vi "binary to msgpack.vi"(11 "binary":u8[](array[numeric])) -> (3 "msgpack":u8[](array[numeric]) format="%x")   [LabVIEW 2020, in "MessagePack.lvlib" / "MessagePack.lvclass"]
uses:
  MessagePack.lvclass
  MessagePack.lvclass/MessagePack.ctl
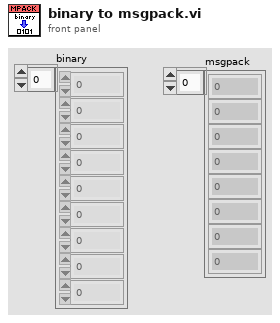
[diagram p1: front panel]
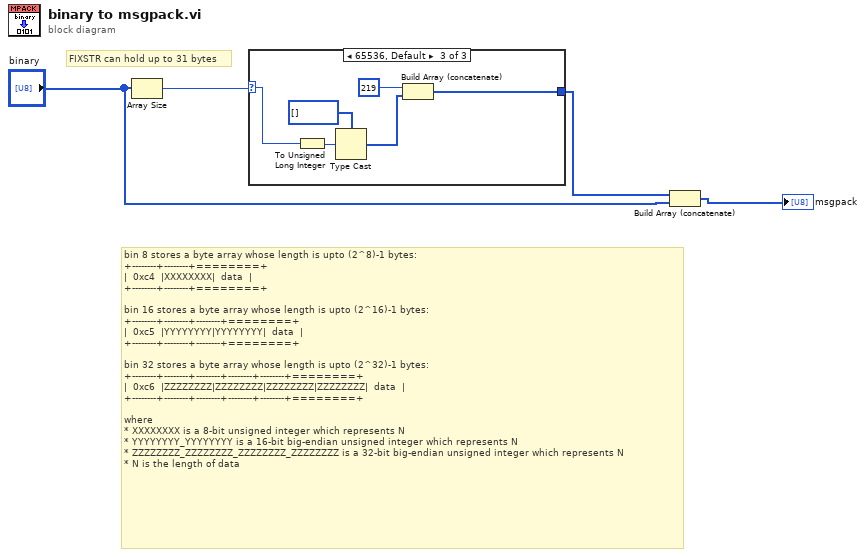
[diagram p0: block diagram]
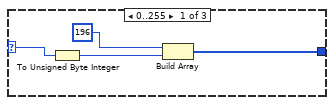
[diagram p2: hidden frame]
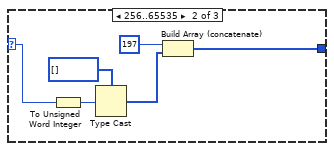
[diagram p3: hidden frame]
diagram:
  # "bin 8 stores a byte array whose length is upto (2^8)-1 bytes:\n+--------+--------+========+\n|  0xc4  |XXXXXXXX|  data  |\n+--------+--------+========+\n\nbin 16 stores a byte array whose length is upto (2^16)-1 bytes:\n+--------+--------+--------+========+\n|  0xc5  |YYYYYYYY|YYYYYYYY|  data  |\n+--------+--------+--------+========+\n\nbin 32 stores a byte array whose length is upto (2^32)-1 bytes:\n+--------+--------+--------+--------+--------+========+\n|  0xc6  |ZZZZZZZZ|ZZZZZZZZ|ZZZZZZZZ|ZZZZZZZZ|  data  |\n+--------+--------+--------+--------+--------+========+\n\nwhere\n* XXXXXXXX is a 8-bit unsigned integer which represents N\n* YYYYYYYY_YYYYYYYY is a 16-bit big-endian unsigned integer which represents N\n* ZZZZZZZZ_ZZZZZZZZ_ZZZZZZZZ_ZZZZZZZZ is a 32-bit big-endian unsigned integer which represents N\n* N is the length of data"
  # "FIXSTR can hold up to 31 bytes"
  n1 = Array Size(array="binary") -> (size(s)=w2:i32)
  n2 = case shown="65536, Default" w2 {
    selector: w2 -> [w8 w12 w15]
    tunnel: [w5 w13 w19] -> w1
    frame 0..255 {
      n3 = To Unsigned Byte Integer(number=w8) -> (unsigned 8bit integer=w6:u8)
      n4 = Build Array(u8 196 ("y"), w6) -> (w5:u8[])
    }
    frame 256..65535 {
      n5 = To Unsigned Word Integer(number=w12) -> (unsigned 16bit integer=w10:u16)
      n6 = Type Cast(type=u8[] [] ("bytes"), x=w10) -> (*(type *) &x=w9:u8[])
      n7 = Build Array (concatenate)(u8 197 ("y"), w9) -> (w13:u8[])
    }
    frame 65536, Default {
      n8 = To Unsigned Long Integer(number=w15) -> (unsigned 32bit integer=w16:u32)
      n9 = Type Cast(type=u8[] [] ("bytes"), x=w16) -> (*(type *) &x=w17:u8[])
      n10 = Build Array (concatenate)(u8 219 ("y"), w17) -> (w19:u8[])
    }
  }
  n11 = Build Array (concatenate)(w1, "binary") -> (→"msgpack":u8[])
